vi "Get Current Target MAC Address2.vi"(8 "error in (no error)":errorcluster) -> (0 "error out":errorcluster, 2 "Clock_ID":string, 3 "MAC address (HEX String)":string)   [LabVIEW 2014]
uses:
  <vilib>/real-time/NI_Real-Time Libraries.lvlib
panel:
  out "length":i32
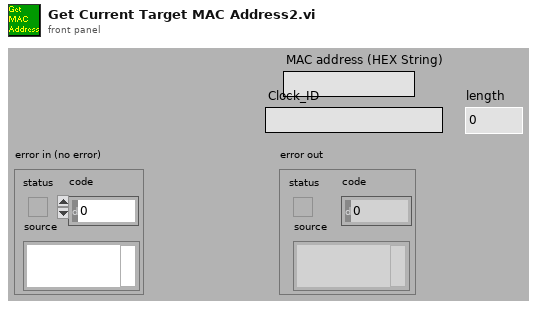
[diagram p1: front panel]
types:
  T1 = cluster{"local subnet?":bool, "IP address":string}
  T2 = cluster{"MAC address":string, "IP address":string, "status":string, "model":string, "Hostname":string}[]
  T3 = cluster{"MAC address":string, "IP address":string, "status":string, "model":string, "Hostname":string}
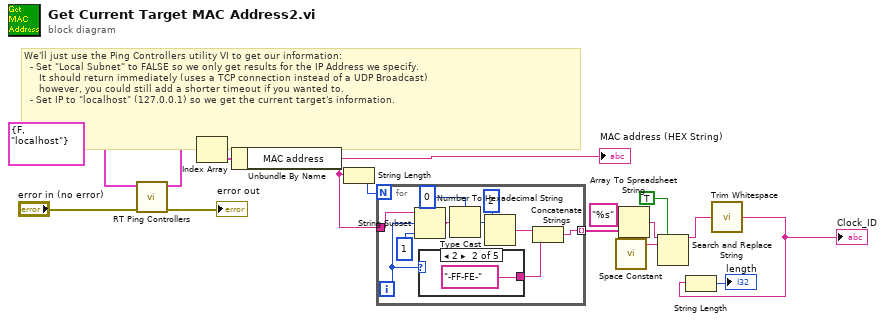
[diagram p0: block diagram]
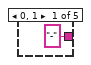
[diagram p2: hidden frame]
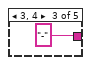
[diagram p3: hidden frame]
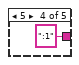
[diagram p4: hidden frame]
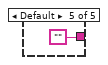
[diagram p5: hidden frame]
diagram:
  # "We'll just use the Ping Controllers utility VI to get our information:\n  - Set \"Local Subnet\" to FALSE so we only get results for the IP Address we specify.  \n     It should return immediately (uses a TCP connection instead of a UDP Broadcast)\n     however, you could still add a shorter timeout if you wanted to.\n  - Set IP to \"localhost\" (127.0.0.1) so we get the current target's information."
  n1 = call <vilib>:"RT Ping Controllers.vi"("error in (no error)"="error in (no error)", "system location (local subnet)"=T1 {"local subnet?"=FALSE, "IP address"="localhost"}) -> ("error out"=→"error out":errorcluster, "Controllers on Subnet"=w12:T2)  [unwired: 8 in]
  n2 = Index Array(array=w12) -> (element=w11:T3)  [unwired: 1 in]
  n3 = Unbundle By Name(w11) -> ("MAC address"=w9:string)
  "MAC address (HEX String)" <- w9
  n4 = String Length(string=w9) -> (length=w10:i32)
  n5 = for {
    N: w10 -> [_]
    tunnel: w9 -> [w25]
    tunnel: [w16] -> w8 mode=indexing
    i -> [w19]
    n6 = String Subset(string=w25, offset (0)=w19, length (rest)=1 ("length (rest)")) -> (substring=w23:string)
    n7 = case shown="2" w19 {
      tunnel: ["-" "-FF-FE-" "-" ":1" ""] -> w17
      frame 0, 1 {
      }
      frame 2 {
      }
      frame 3, 4 {
      }
      frame 5 {
      }
      frame Default {
      }
    }
    n8 = Type Cast(type=u8 0, x=w23) -> (*(type *) &x=w21:u8)
    n9 = Number To Hexadecimal String(1:i16 2 ("width (-)"), 2:w21) -> (0:w18:string)
    n10 = Concatenate Strings(w18, w17) -> (w16:string)
  }
  n11 = call <vilib>:"Space Constant.vi"() -> ("String"=w5:string)
  n12 = Array To Spreadsheet String(delimiter (Tab)=w5, array=w8, 3:"%s" ("format string")) -> (spreadsheet string=w6:string)
  n13 = Search and Replace String(replace all?=TRUE ("replace all? (F)"), input string=w6, search string=w5) -> (result string=w2:string)  [unwired: 5 in, 3 out]
  n14 = call <vilib>:"Trim Whitespace.vi"("string"=w2) -> ("trimmed string"=w1:string)  [unwired: 1 in]
  "Clock_ID" <- w1
  n15 = String Length(string=w1) -> (length=→"length":i32)
